vi "Serialize to JSON.vi"(8 "error in (no error)":errorcluster, 11 "Pkg Details in":refnum<class "Package Version.lvclass">) -> (0 "error out":errorcluster, 1 "JSON Value":refnum<class "JSON Value.lvclass">, 2 "JSON string":string, 3 "Pkg Details out":refnum<class "Package Version.lvclass">)   [LabVIEW 2016, in "Packages.lvlib" / "Package Version.lvclass"]
uses:
  Package Version.lvclass
  <vilib>/addons/JSON API/JSON Value/JSON Value.lvclass
  Package Version.lvclass/Package Version.ctl
  <vilib>/addons/JSON API/Variant JSON/Variant JSON.lvlib
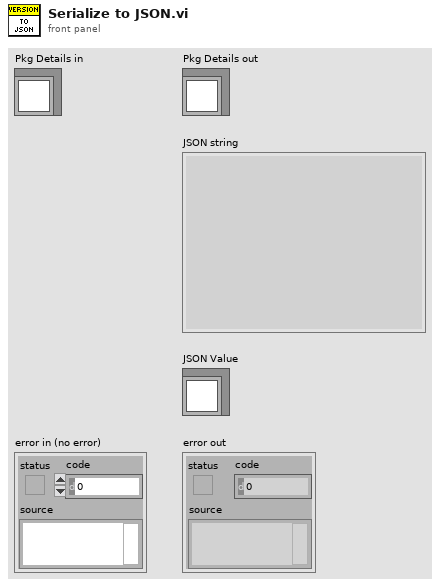
[diagram p1: front panel]
types:
  T1 = typedef "Packages.lvlib/Repo.lvclass/RepoType--enum.ctl" = enum16{"VIPM", "NIPM", "GPM"}
  T2 = cluster{"ReleaseDate":timestamp, "Version":string, "Name":string, "DisplayName":string, "Description":string, "Vendor":string, "Author":string, "Release Notes":string, "Dependencies":string[], "IconURL":string, "PackageURL":string, "RepoType":T1, "RepoName":string}
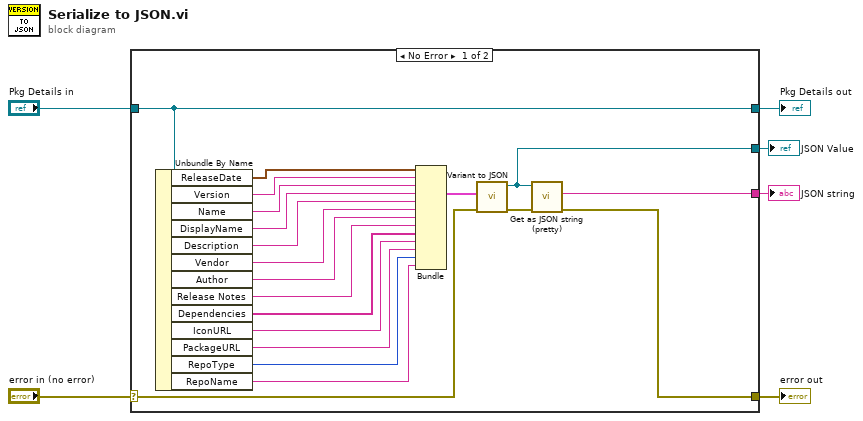
[diagram p0: block diagram]
diagram:
  n1 = case shown="No Error" "error in (no error)" {
    selector: "error in (no error)" -> [w26 w28]
    tunnel: [w18 w28] -> w5
    tunnel: [w25 w27] -> w3
    tunnel: "Pkg Details in" -> [w25 w27]
    tunnel: [w16 _] -> w2
    tunnel: [w15 _] -> w1
    frame No Error {
      n2 = Unbundle By Name(w25) -> ("ReleaseDate"=w14:timestamp, "Version"=w13:string, "Name"=w9:string, "DisplayName"=w10:string, "Description"=w24:string, "Vendor"=w23:string, "Author"=w22:string, "Release Notes"=w21:string, "Dependencies"=w20:string[], "IconURL"=w12:string, "PackageURL"=w11:string, "RepoType"=w8:T1, "RepoName"=w7:string)
      n3 = Bundle("ReleaseDate"=w14, "Version"=w13, "Name"=w9, "DisplayName"=w10, "Description"=w24, "Vendor"=w23, "Author"=w22, "Release Notes"=w21, "Dependencies"=w20, "IconURL"=w12, "PackageURL"=w11, "RepoType"=w8, "RepoName"=w7) -> (w17:T2)  [unwired: 1 in]
      n4 = call <vilib>:"Variant to JSON.vi"("error in (no error)"=w26, "Variant"=w17) -> ("error out"=w19:errorcluster, "JSON Value out"=w15:refnum<class "JSON Value.lvclass">)  [unwired: 8 in]
      n5 = call <vilib>:"Get as JSON string (pretty).vi"("error in (no error)"=w19, "JSON Value in"=w15) -> ("error out"=w18:errorcluster, "<JSON>"=w16:string)  [unwired: 8 in]
    }
    frame Error {
    }
  }
  "error out" <- w5
  "Pkg Details out" <- w3
  "JSON string" <- w2
  "JSON Value" <- w1
